vi "ARINC to Hex converter.vi"() -> ()   [LabVIEW 2012]
uses:
  RT/Typdefs/ARINC word.ctl
panel:
  out "Numeric":u32 format="%.0x"
  in  "ARINC word in":T1 format="%032b"
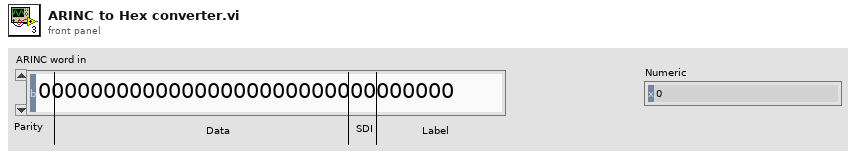
[diagram p1: front panel]
types:
  T1 = typedef "ARINC word.ctl" = u32
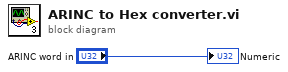
[diagram p0: block diagram]
diagram:
  "Numeric" <- "ARINC word in"
